vi "Keywords Log file.vi"(8 "error in (no error)":errorcluster) -> (0 "error in (no error) 2":errorcluster)   [LabVIEW 2018]
uses:
  <vilib>/addons/_JKI Toolkits/Caraya/classes/Test/Test.lvclass
  Log File/CCS_Log File.lvclass
  <vilib>/addons/_JKI Toolkits/Caraya/classes/Assert/Assert.lvclass
  <vilib>/addons/_JKI Toolkits/Caraya/classes/Assert/Assert Equal Value_Variant.vi
  Keywords Log File/Keywords Log File.lvclass
  C:/Users/Denis/Desktop/S4CCS/S4CCS/Log File/CCS_Log File.lvclass
  <vilib>/addons/_JKI Toolkits/Caraya/classes/Assert/Assert Not Error.vi
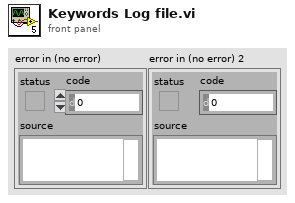
[diagram p1: front panel]
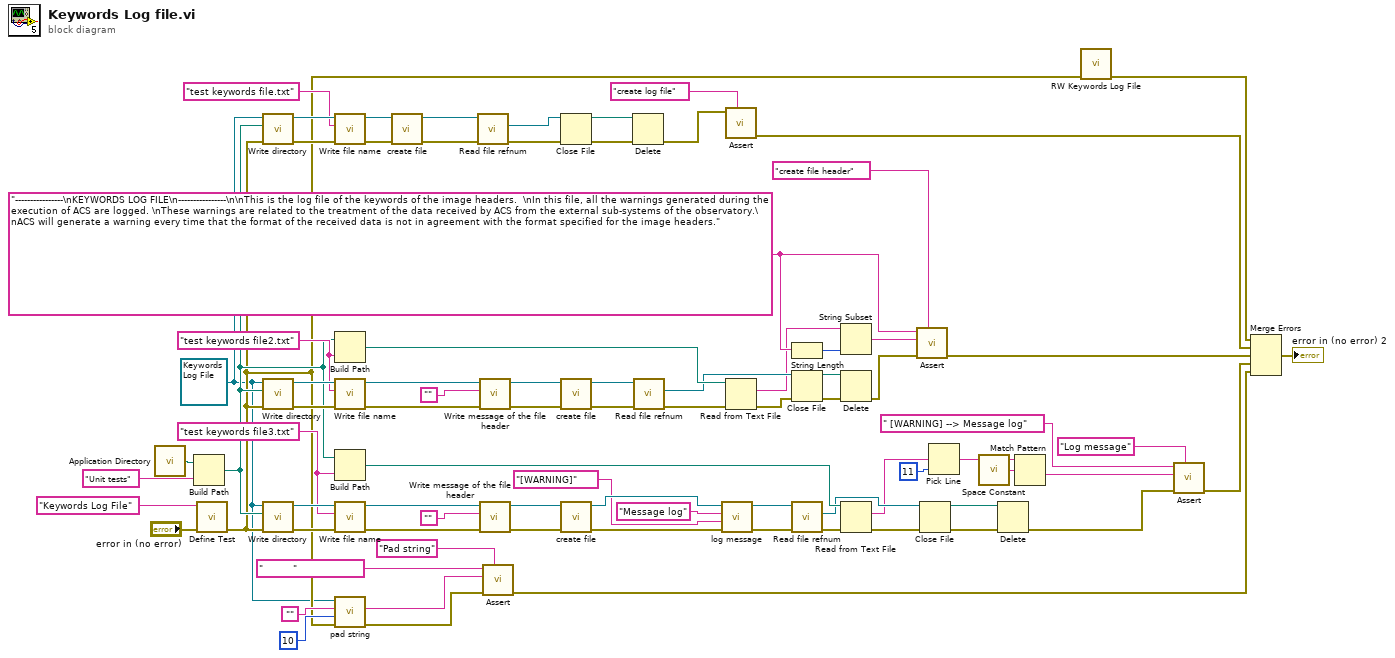
[diagram p0: block diagram]
diagram:
  w5 = refnum<class "Keywords Log File.lvclass"> refnum ("Keywords Log File.lvclass")
  w31 = "test keywords file3.txt" ("file name")
  w4 = "----------------\nKEYWORDS LOG FILE\n----------------\n\nThis is the log file of the keywords of the image headers.  \nIn this file, all the warnings generated during the execution of ACS are logged. \nThese warnings are related to the treatment of the data received by ACS from the external sub-systems of the observatory.\nACS will generate a warning every time that the format of the received data is not in agreement with the format specified for the image headers." ("Label (VI Title)")
  w53 = "test keywords file2.txt" ("file name")
  n1 = call <vilib>:"Application Directory.vi"() -> ("Application Directory"=w76:path)
  n2 = Build Path(base path=w76, name or relative path="Unit tests") -> (appended path=w30:path)
  n3 = call <vilib>:"Define Test.vi"("error in (no error)"="error in (no error)", "Label (VI Title)"="Keywords Log File") -> ("error out"=w6:errorcluster)  [unwired: 8 in, 1 out]
  n4 = call "Write directory.vi"("error in (no error)"=w6, 10:w30, "Log File in"=w5) -> ("error out"=w78:errorcluster, "Log File out"=w77:refnum<class "Keywords Log File.lvclass">)  [unwired: 7 in]
  n5 = call "Write directory.vi"("error in (no error)"=w6, 10:w30, "Log File in"=w5) -> ("error out"=w62:errorcluster, "Log File out"=w61:refnum<class "Keywords Log File.lvclass">)  [unwired: 7 in]
  n6 = call "Write directory.vi"("error in (no error)"=w6, 10:w30, "Log File in"=w5) -> ("error out"=w41:errorcluster, "Log File out"=w40:refnum<class "Keywords Log File.lvclass">)  [unwired: 7 in]
  n7 = call "Write file name.vi"("error in (no error)"=w78, "file name"="test keywords file.txt", "Log File in"=w77) -> ("error out"=w63:errorcluster, "Log File out"=w64:refnum<class "Keywords Log File.lvclass">)  [unwired: 7 in]
  n8 = Build Path(base path=w30, name or relative path=w53) -> (appended path=w52:path)
  n9 = call "Write file name.vi"("error in (no error)"=w62, "file name"=w53, "Log File in"=w61) -> ("error out"=w57:errorcluster, "Log File out"=w60:refnum<class "Keywords Log File.lvclass">)  [unwired: 7 in]
  n10 = Build Path(base path=w30, name or relative path=w31) -> (appended path=w32:path)
  n11 = call "Write file name.vi"("error in (no error)"=w41, "file name"=w31, "Log File in"=w40) -> ("error out"=w44:errorcluster, "Log File out"=w39:refnum<class "Keywords Log File.lvclass">)  [unwired: 7 in]
  n12 = call "pad string.vi"("error in (no error)"=w6, "string size"=u16 10, "input string"="", "Log File in"=w5) -> ("error out"=w7:errorcluster, "output string"=w11:string)  [unwired: 5 in, 1 out]
  n13 = call "create file.vi"("error in (no error)"=w63, "Log File in"=w64) -> ("error out"=w66:errorcluster, "Log File out"=w65:refnum<class "Keywords Log File.lvclass">)  [unwired: 8 in]
  n14 = call "Read file refnum.vi"("error in (no error)"=w66, "Log File in"=w65) -> ("error out"=w70:errorcluster, "file refnum"=w67:refnum<file>)  [unwired: 7 in, 1 out]
  n15 = call "Write message of the file header.vi"("error in (no error)"=w57, "message of the file header"="", "Log File in"=w60) -> ("error out"=w58:errorcluster, "Log File out"=w59:refnum<class "Keywords Log File.lvclass">)  [unwired: 7 in]
  n16 = call "Write message of the file header.vi"("error in (no error)"=w44, "message of the file header"="", "Log File in"=w39) -> ("error out"=w43:errorcluster, "Log File out"=w38:refnum<class "Keywords Log File.lvclass">)  [unwired: 7 in]
  n17 = call-poly <vilib>:"Assert.vi"("Label"="Pad string" ("Label (VI Title)"), "error in (no error)"=w7, "Y"=w11, "X"="          ") -> ("error out"=w8:errorcluster)  [unwired: 6 in, 1 out]
  n18 = Close File(refnum=w67, error in=w70) -> (path=w68:path, error out=w69:errorcluster)
  n19 = call "create file.vi"("error in (no error)"=w58, "Log File in"=w59) -> ("error out"=w56:errorcluster, "Log File out"=w55:refnum<class "Keywords Log File.lvclass">)  [unwired: 8 in]
  n20 = call "create file.vi"("error in (no error)"=w43, "Log File in"=w38) -> ("error out"=w42:errorcluster, "Log File out"=w35:refnum<class "Keywords Log File.lvclass">)  [unwired: 8 in]
  n21 = Delete(path (use dialog)=w68, error in=w69) -> (error out=w74:errorcluster)  [unwired: 3 in, 2 out]
  n22 = call "Read file refnum.vi"("error in (no error)"=w56, "Log File in"=w55) -> ("error out"=w54:errorcluster, "file refnum"=w45:refnum<file>)  [unwired: 7 in, 1 out]
  n23 = call-dynamic "log message.vi"("error in (no error)"=w42, "message type"="[WARNING]", "Message to log"="Message log", "Log File in"=w35) -> ("error out"=w21:errorcluster, "Log File out"=w20:refnum<class "Keywords Log File.lvclass">)  [unwired: 6 in]
  n24 = call-poly <vilib>:"Assert.vi"("Label"="create log file" ("Label (VI Title)"), "Not Error?"=w74) -> ("error out"=w73:errorcluster)  [unwired: 8 in, 1 out]
  n25 = Read from Text File(file (use dialog)=w52, error in=w54) -> (text=w2:string, error out=w49:errorcluster)  [unwired: 2 in, 2 out]
  n26 = String Length(string=w4) -> (length=w3:i32)
  n27 = Close File(refnum=w45, error in=w49) -> (path=w47:path, error out=w50:errorcluster)
  n28 = call "Read file refnum.vi"("error in (no error)"=w21, "Log File in"=w20) -> ("error out"=w19:errorcluster, "file refnum"=w18:refnum<file>)  [unwired: 7 in, 1 out]
  n29 = String Subset(string=w2, length (rest)=w3) -> (substring=w1:string)  [unwired: 1 in]
  n30 = Delete(path (use dialog)=w47, error in=w50) -> (error out=w48:errorcluster)  [unwired: 3 in, 2 out]
  n31 = Read from Text File(file (use dialog)=w32, error in=w19) -> (text=w15:string, error out=w27:errorcluster)  [unwired: 2 in, 2 out]
  n32 = call-poly <vilib>:"Assert.vi"("Label"="create file header" ("Label (VI Title)"), "error in (no error)"=w48, "Y"=w1, "X"=w4) -> ("error out"=w51:errorcluster)  [unwired: 6 in, 1 out]
  n33 = Close File(refnum=w18, error in=w27) -> (path=w29:path, error out=w28:errorcluster)
  n34 = Pick Line(multi-line string=w15, line index=11) -> (output string=w16:string)  [unwired: 1 in]
  n35 = call <vilib>:"Space Constant.vi"() -> ("String"=w22:string)
  n36 = Delete(path (use dialog)=w29, error in=w28) -> (error out=w25:errorcluster)  [unwired: 3 in, 2 out]
  n37 = Match Pattern(string=w16, regular expression=w22) -> (after substring=w23:string)  [unwired: 1 in, 3 out]
  n38 = call "RW Keywords Log File.vi"("error in (no error)"=w6) -> ("error in (no error) 2"=w79:errorcluster)  [unwired: 10 in]
  n39 = call-poly <vilib>:"Assert.vi"("Label"="Log message" ("Label (VI Title)"), "error in (no error)"=w25, "Y"=w23, "X"=" [WARNING] --> Message log" ("Label (VI Title)")) -> ("error out"=w26:errorcluster)  [unwired: 6 in, 1 out]
  n40 = Merge Errors(w79, w73, w51, w26, w8) -> (→"error in (no error) 2":errorcluster)
